vi "Acquisition Integer Low Rate Test.vi"   [LabVIEW 2014]
uses:
  <vilib>/Platform/TimedLoop/XDataNode/timing_clust.ctl
  <vilib>/Platform/TimedLoop/XDataNode/nitl_modes.ctl
  <vilib>/Platform/TimedLoop/XDataNode/wakeup.ctl
  <vilib>/rvi/eio/common/nirviEmuTemplateMethod_errors.vi
  <vilib>/rvi/Emulation/niFpgaSctlEmulationGetInTimedLoop.vi
  <vilib>/rvi/Emulation/niFpgaEmulationReportErrorSimple.vi
  <vilib>/rvi/Emulation/niFpgaGetClockAttributes.vi
  <vilib>/rvi/Emulation/niFpgaCriticalErrorInLSC.vi
  <vilib>/rvi/interface/RandomDataEmulation/niFpgaRandomDataHandleErrors.vi
  <vilib>/Platform/TimedLoop/XDataNode/XDataNode.xnode
  <vilib>/eio/EIOMethodNode/EIOMethodNode.xnode
  <vilib>/rvi/DataTransferAndStorage/Container/XNode/niFpgaContainer.xnode
  <vilib>/rvi/interface/RandomDataEmulation/nirviRandomDataFpgaReadWriteTemplate.vi
  <vilib>/Platform/TimedLoop/XDataNode/XDNodeRunTimeDep.lvlib
types:
  T1 = typedef "XDNodeRunTimeDep.lvlib/timing_clust.ctl" = cluster{"Expected End [f-1]":u64, "Actual End [f-1]":u64, "Finished Late? [f-1]":bool, "Expected End [i-1]":u64, "Actual End [i-1]":u64, "Finished Late? [i-1]":bool, "Expected Start [i]":u64, "Actual Start [i]":u64, "Expected Start [f]":u64, "Actual Start [f]":u64, "Source Name":string, "Structure Name":string, "Period":i64, "Deadline":i64, "Offset":i64, "Start":i64, "Priority":i32, "Timeout":i32, "Mode":T2, "Wakeup Reason":T3, "Error":errorcluster, "Source Type":string, "Secondary Source Type":string, "Global End Time":u64, "Global Start Time":u64, "Frame Duration":u64, "Iteration Duration":u64, "Assigned CPU":i32, "I/O Scan Engine Mode":u32}
  T2 = typedef "XDNodeRunTimeDep.lvlib/nitl_modes.ctl" = enum32{"No Change", "Process missed periods, maintain original phase", "Discard missed periods, maintain original phase", "Process missed periods, ignore original phase", "Discard missed periods, ignore original phase"}
  T3 = typedef "XDNodeRunTimeDep.lvlib/wakeup.ctl" = enum32{"Normal", "Aborted", "Asynchronous wakeup", "Timing source error", "Timed loop error", "Timeout"}
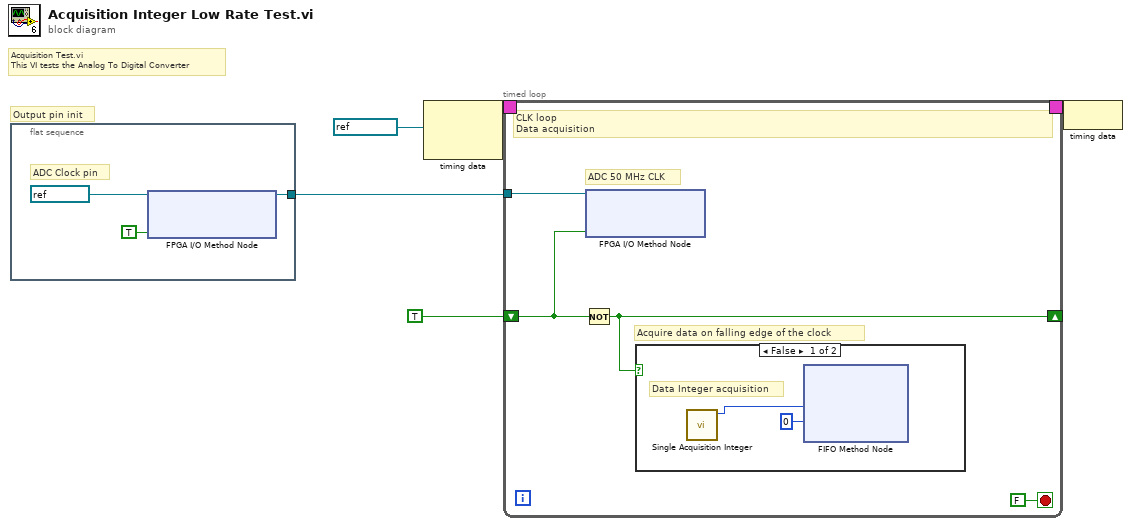
[diagram p0: block diagram]
diagram:
  # "Acquisition Test.vi\nThis VI tests the Analog To Digital Converter"
  # "Output pin init"
  n1 = flat-sequence {
    tunnel: [w6] -> w1
    frame #0 {
      # "ADC Clock pin"
      n2 = xnode "FPGA I/O Method Node"("FPGA I/O In"=refnum<k21> "DIO17", "Enable"=TRUE) -> ("FPGA I/O Out"=w6:refnum<k21>)
    }
  }
  n3 = node-c288(refnum<k21> "2.5MHz" ("Source Name")) -> (w5:T1)  [unwired: 1 in]
  n4 = timed-loop {
    timing: w5 -> [_]
    timing-out: [_] -> w4
    shift-right: [w10] -> _
    shift-left: TRUE -> [w9]
    tunnel: w1 -> [w12]
    stop <- FALSE stop-if-true
    # "Acquire data on falling edge of the clock"
    # "ADC 50 MHz CLK"
    # "CLK loop\nData acquisition"
    n5 = Not(x=w9) -> (.not. x?=w10:bool)
    n6 = xnode "FPGA I/O Method Node"("FPGA I/O In"=w12, "Data"=w9) -> ()  [unwired: 1 out]
    n7 = case shown="False" w10 {
      frame False {
        # "Data Integer acquisition"
        n8 = call "Single Acquisition Integer.vi"() -> ("number"=w13:u16)  [unwired: 11 in]
        n9 = xnode ("FIFO Method Node")("Element"=w13, "Timeout"=0) -> ()  [unwired: 1 in, 2 out]
      }
      frame True {
      }
    }
  }
  n10 = node-c288(w4) -> ()
